vi "ASrreglo2dispINIC.vi"(8 "dimension adqy":i32=2, 9 "dimension adqx":i32=6, 10 "dimension disp 2":i32=3, 11 "dimension disp 1":i32=5) -> (2 "output array":dbl[][][][](array[numeric]))   [LabVIEW 2016]
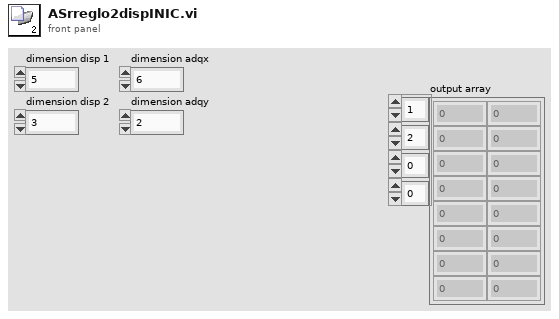
[diagram p1: front panel]
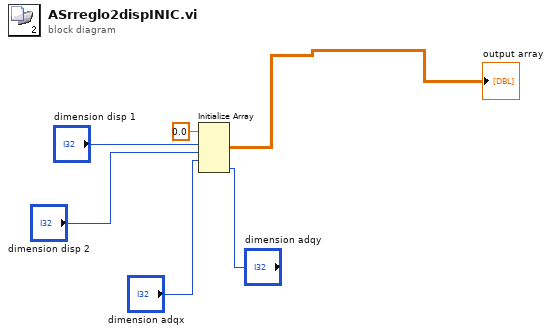
[diagram p0: block diagram]
diagram:
  n1 = Initialize Array(0.0 ("element"), "dimension disp 1", "dimension disp 2", "dimension adqx", "dimension adqy") -> (→"output array":dbl[][][][])
